vi "Nov_30.vi"() -> ()   [LabVIEW 2020]
uses:
  <vilib>/Analysis/3filter.llb/Filter Passband Type.ctl
  <vilib>/DAQmx/read.llb/DAQmx Read (Analog 1D DBL NChan 1Samp).vi
  <vilib>/DAQmx/create/channels.llb/DAQmx Create Channel (AI-Voltage-Basic).vi
  <vilib>/DAQmx/miscellaneous.llb/DAQmx Fill In Error Info.vi
  <vilib>/Analysis/3filter.llb/Butterworth Filter (DBL).vi
  <vilib>/Utility/file.llb/Write Delimited Spreadsheet (string).vi
  <vilib>/Utility/file.llb/Write Delimited Spreadsheet (DBL).vi
  <vilib>/Analysis/NI_AALBase.lvlib
panel:
  out "Force Plate":dynamicdata(graph)
  out "Swing":bool
  out "Accelerometers":dynamicdata(graph)
  out "Hit 1":bool
  out "Enlapsed Time (sec)":dbl
  in  "stop":bool
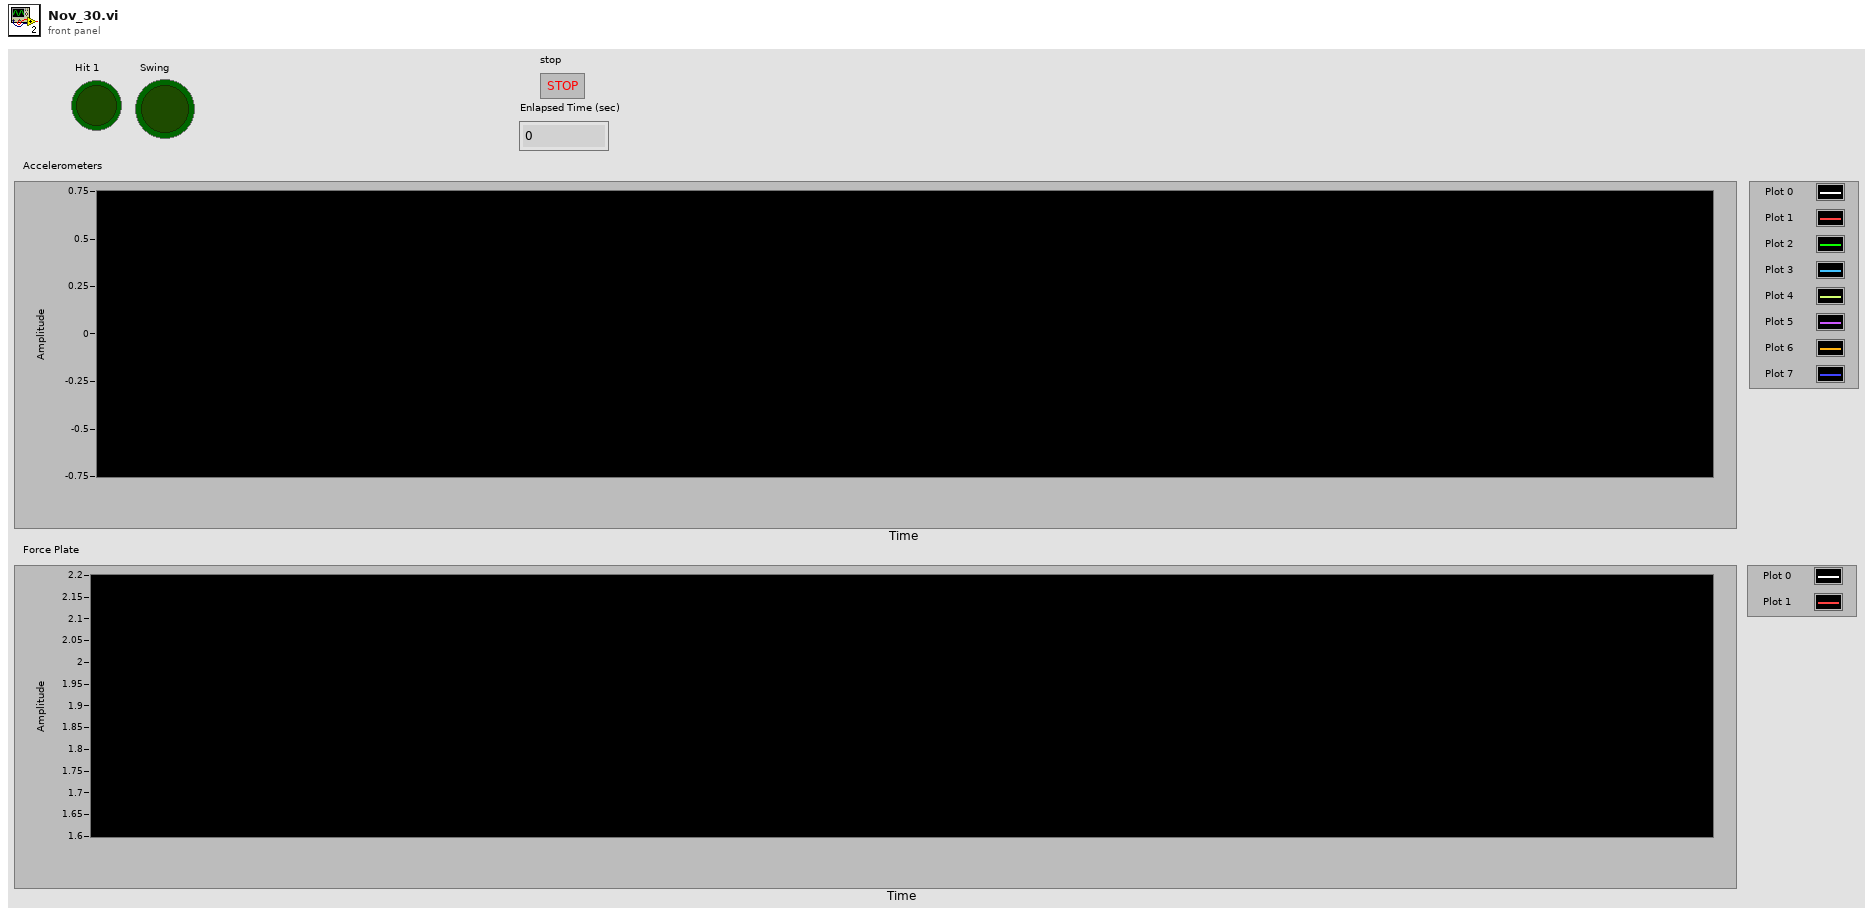
[diagram p1: front panel]
types:
  T1 = typedef "NI_AALBase.lvlib/Filter Passband Type.ctl" = enum32{"Lowpass", "Highpass", "Bandpass", "Bandstop"}
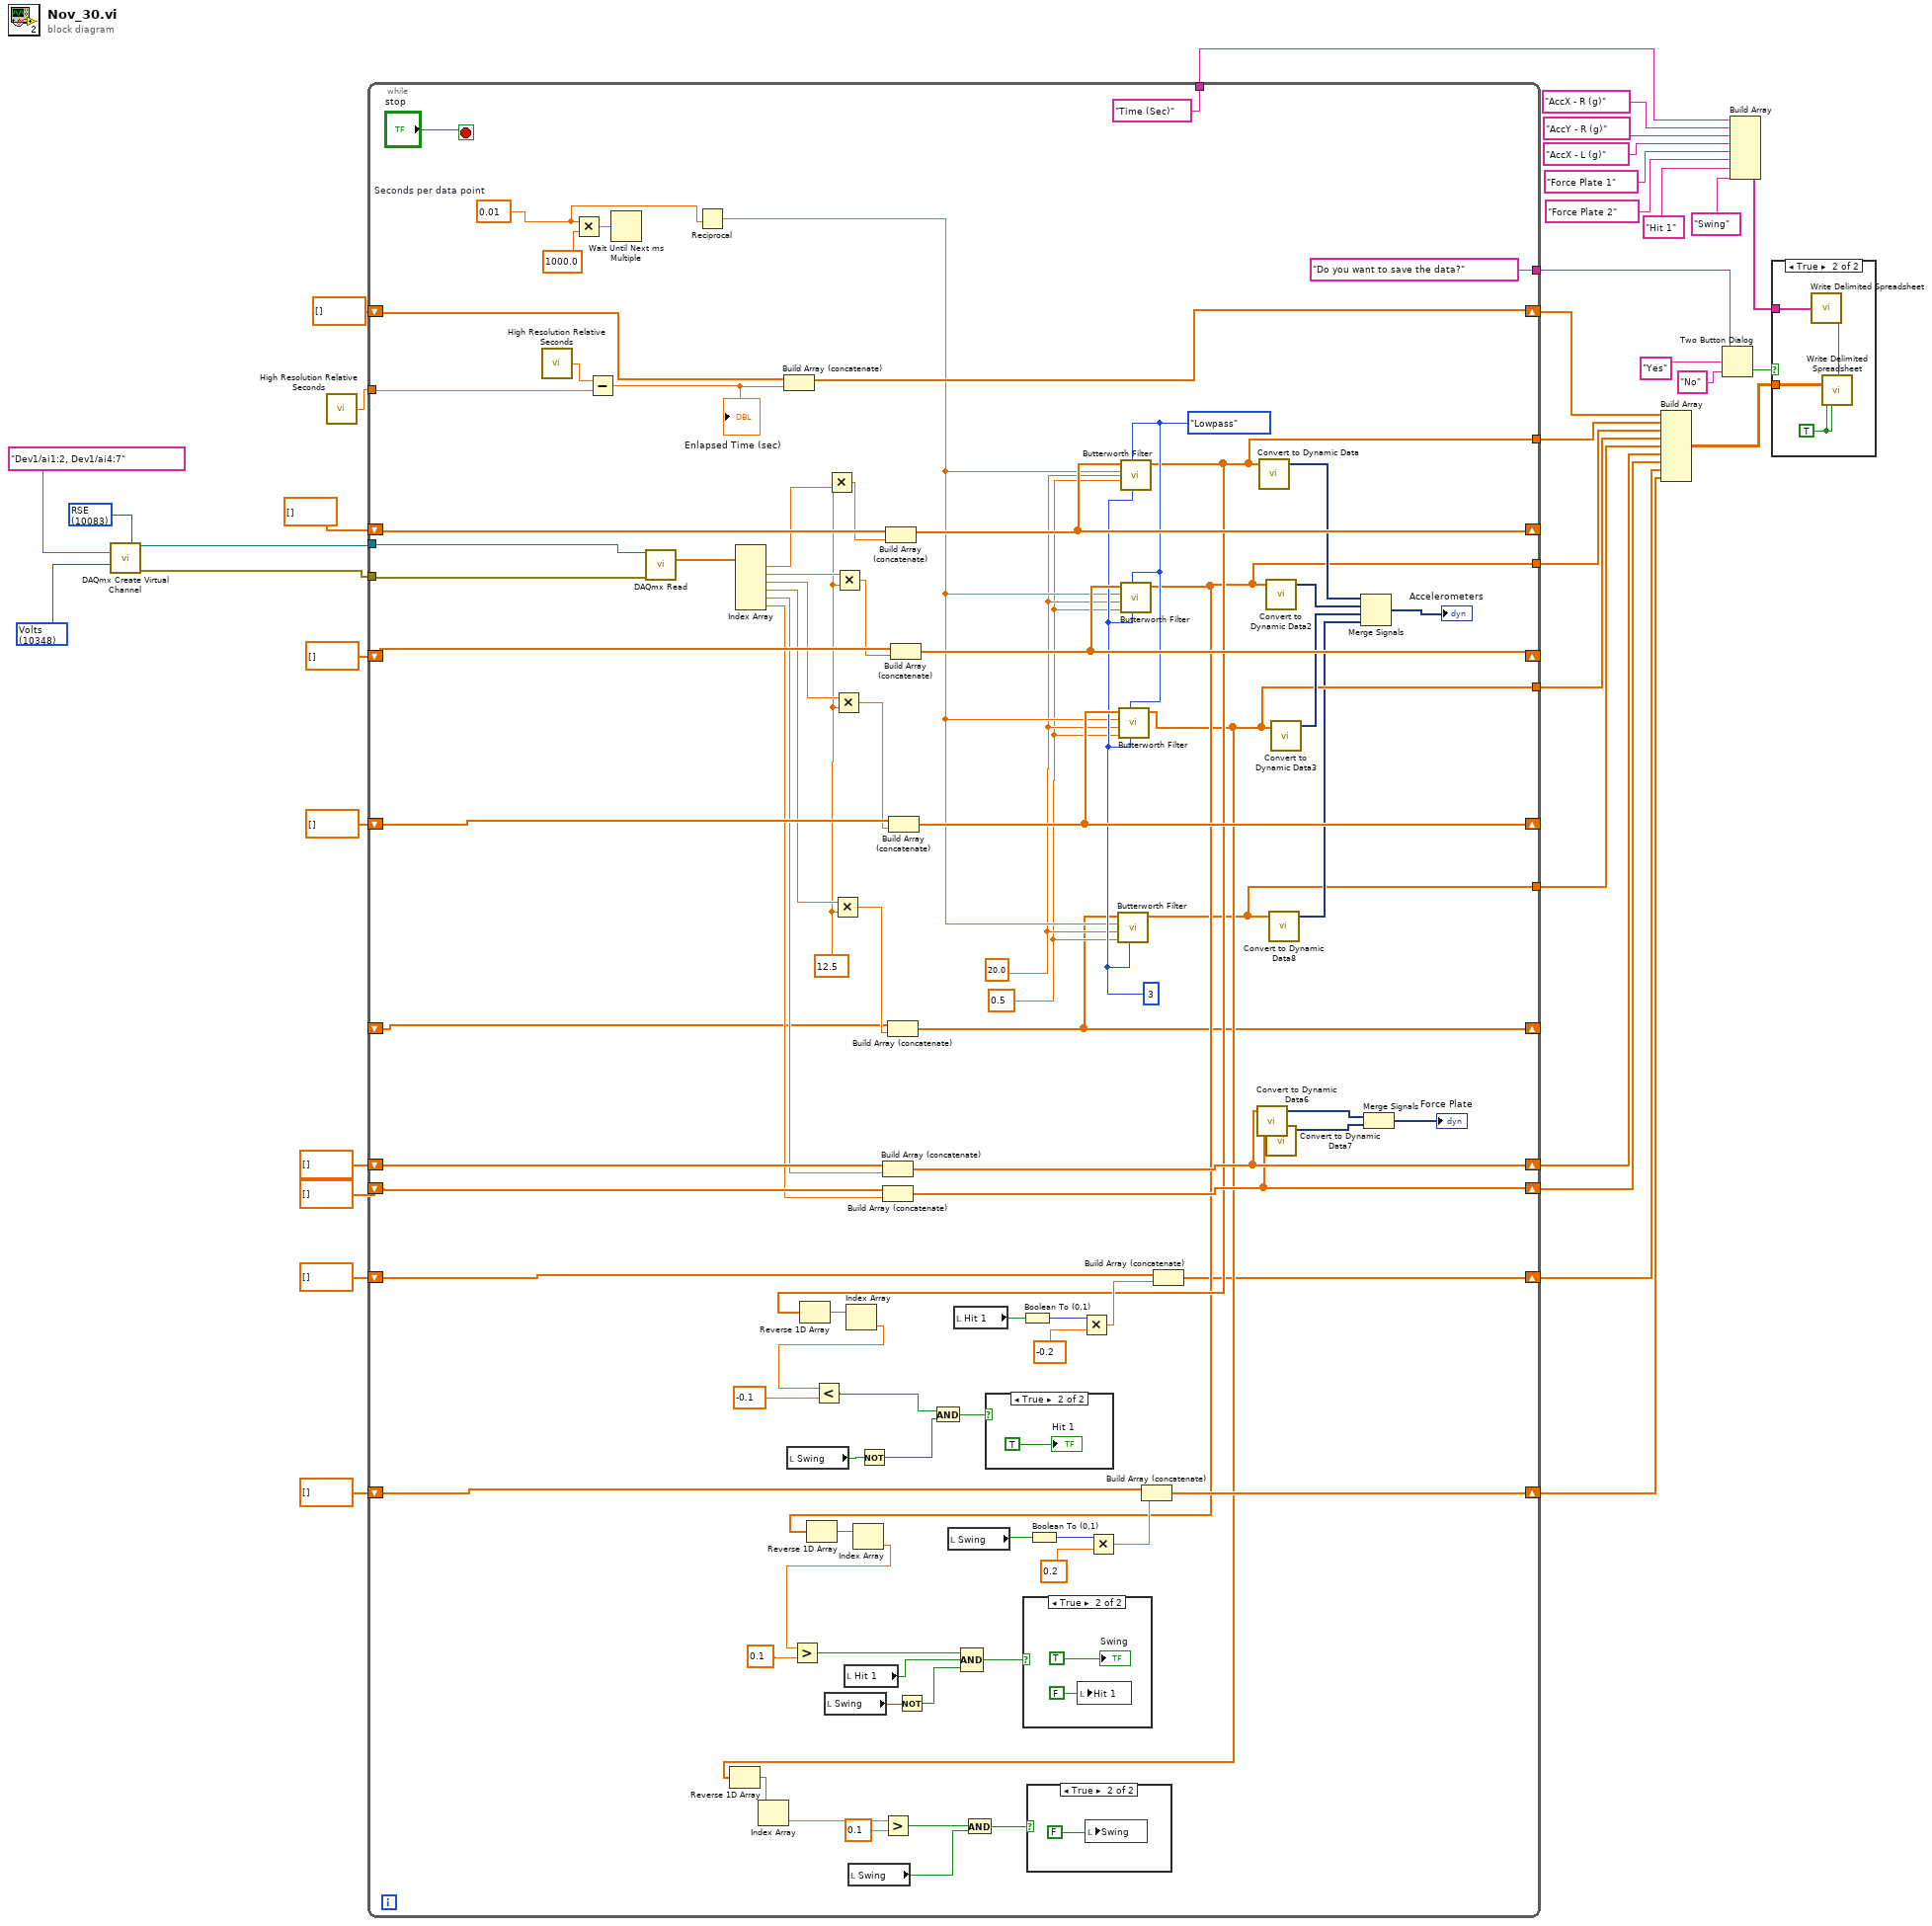
[diagram p0: block diagram]
diagram:
  w20 = 10348 items=["Volts"=10348, "From Custom Scale"=10065] ("units")
  w21 = 10083 items=["Default"=-1, "RSE"=10083, "NRSE"=10078, "Differential"=10106, "Pseudodifferential"=12529] ("input terminal configuration")
  n1 = call-poly <vilib>:"DAQmx Create Virtual Channel.vi"("input terminal configuration"=w21, "physical channels"=tag "Dev1/ai1:2, Dev1/ai4:7" ("Physical channels"), "units"=w20) -> ("task out"=w23:refnum<k21>, "error out"=w24:errorcluster)  [unwired: 11 in]
  n2 = call <vilib>:"High Resolution Relative Seconds.vi"() -> ("relative seconds"=w37:dbl)
  n3 = while {
    tunnel: w23 -> [w124]
    tunnel: w24 -> [w123]
    tunnel: w37 -> [w118]
    shift-right: [w83] -> w34
    shift-left: dbl[] [] -> [w116]
    shift-right: [w101] -> _
    shift-left: dbl[] [] -> [w114]
    shift-right: [w100] -> _
    shift-left: dbl[] [] -> [w113]
    tunnel: ["Time (Sec)"] -> w29
    tunnel: ["Do you want to save the data?" ("message")] -> w25
    shift-right: [w38] -> w4
    shift-left: dbl[] [] -> [w107]
    shift-right: [w79] -> w5
    shift-left: dbl[] [] -> [w90]
    shift-right: [w84] -> _
    shift-left: dbl[] [] -> [w87]
    shift-right: [w58] -> w2
    shift-left: dbl[] [] -> [w61]
    shift-right: [w56] -> w3
    shift-left: dbl[] [] -> [w60]
    tunnel: [w54] -> w8
    tunnel: [w53] -> w7
    tunnel: [w52] -> w6
    shift-right: [w41] -> _
    shift-left: _ -> [w40]
    tunnel: [w39] -> w1
    stop <- "stop" stop-if-true
    w48 = 3 ("order")
    w45 = 0.5 ("low cutoff freq: fl")
    w46 = 20.0 ("high cutoff freq: fh")
    w43 = 12.5 ("x")
    w62 = 0.01  # Seconds per data point
    w85 = Filter_Passband_Type."Lowpass" ("filter type")
    n4 = call <vilib>:"High Resolution Relative Seconds.vi"() -> ("relative seconds"=w119:dbl)
    n5 = Multiply(x=w62, y=1000.0) -> (x*y=w121:dbl)
    n6 = Subtract(x=w119, y=w118) -> (x-y=w117:dbl)
    "Enlapsed Time (sec)" <- w117
    n7 = Wait Until Next ms Multiple(millisecond multiple=w121) -> ()  [unwired: 1 out]
    n8 = call-poly <vilib>:"DAQmx Read.vi"("task/channels in"=w124, "error in"=w123) -> ("data"=w115:dbl[])  [unwired: 11 in, 2 out]
    n9 = Reciprocal(x=w62) -> (1/x=w47:dbl)
    n10 = Index Array(array=w115) -> (element #1=w110:dbl, element #2=w108:dbl, element #3=w88:dbl, element #4=w44:dbl, element #5=w50:dbl, element #6=w51:dbl)  [unwired: 6 in]
    n11 = Build Array (concatenate)(w116, w117) -> (w83:dbl[])
    n12 = local read "Swing"() -> (w73:bool)
    n13 = local read "Swing"() -> (w76:bool)
    n14 = Multiply(x=w43, y=w110) -> (x*y=w103:dbl)
    n15 = Multiply(x=w44, y=w43) -> (x*y=w49:dbl)
    n16 = Multiply(x=w88, y=w43) -> (x*y=w86:dbl)
    n17 = Multiply(x=w108, y=w43) -> (x*y=w109:dbl)
    n18 = local read "Hit 1"() -> (w77:bool)
    n19 = local read "Swing"() -> (w66:bool)
    n20 = Not(x=w73) -> (.not. x?=w72:bool)
    n21 = Build Array (concatenate)(w61, w50) -> (w58:dbl[])
    n22 = Build Array (concatenate)(w60, w51) -> (w56:dbl[])
    n23 = Build Array (concatenate)(w114, w103) -> (w101:dbl[])
    n24 = Build Array (concatenate)(w40, w49) -> (w41:dbl[])
    n25 = Build Array (concatenate)(w87, w86) -> (w84:dbl[])
    n26 = Build Array (concatenate)(w113, w109) -> (w100:dbl[])
    n27 = Not(x=w76) -> (.not. x?=w75:bool)
    n28 = local read "Swing"() -> (w89:bool)
    n29 = local read "Hit 1"() -> (w92:bool)
    n30 = Boolean To (0,1)(Boolean=w92) -> (0, 1=w105:i16)
    n31 = Boolean To (0,1)(Boolean=w89) -> (0, 1=w98:i16)
    n32 = Multiply(x=w105, y=-0.2) -> (x*y=w106:dbl)
    n33 = Multiply(x=w98, y=0.2) -> (x*y=w91:dbl)
    n34 = call-poly <vilib>:"Butterworth Filter.vi"("order"=w48, "low cutoff freq: fl"=w45, "high cutoff freq: fh"=w46, "sampling freq: fs"=w47, "X"=w41) -> ("Filtered X"=w39:dbl[])  [unwired: 3 in, 1 out]
    n35 = call-poly <vilib>:"Butterworth Filter.vi"("order"=w48, "filter type"=w85, "low cutoff freq: fl"=w45, "high cutoff freq: fh"=w46, "sampling freq: fs"=w47, "X"=w84) -> ("Filtered X"=w52:dbl[])  [unwired: 2 in, 1 out]
    n36 = Reverse 1D Array(array=w52) -> (reversed array=w64:dbl[])
    n37 = Index Array(array=w64) -> (element=w63:dbl)  [unwired: 1 in]
    n38 = Greater?(x=w63, y=0.1) -> (0:w65:bool)
    n39 = And(x=w65, y=w66) -> (x .and. y?=w67:bool)
    n40 = case shown="True" w67 {
      frame False {
      }
      frame True {
        n41 = local write "Swing"(FALSE) -> ()
      }
    }
    n42 = call-poly <vilib>:"Butterworth Filter.vi"("order"=w48, "filter type"=w85, "low cutoff freq: fl"=w45, "high cutoff freq: fh"=w46, "sampling freq: fs"=w47, "X"=w101) -> ("Filtered X"=w54:dbl[])  [unwired: 2 in, 1 out]
    n43 = Reverse 1D Array(array=w54) -> (reversed array=w102:dbl[])
    n44 = Index Array(array=w102) -> (element=w94:dbl)  [unwired: 1 in]
    n45 = Less?(x=w94, y=-0.1) -> (x < y?=w71:bool)
    n46 = And(x=w71, y=w72) -> (x .and. y?=w70:bool)
    n47 = case shown="True" w70 {
      frame False {
      }
      frame True {
        "Hit 1" <- TRUE
      }
    }
    n48 = call-poly <vilib>:"Butterworth Filter.vi"("order"=w48, "filter type"=w85, "low cutoff freq: fl"=w45, "high cutoff freq: fh"=w46, "sampling freq: fs"=w47, "X"=w100) -> ("Filtered X"=w53:dbl[])  [unwired: 2 in, 1 out]
    n49 = Reverse 1D Array(array=w53) -> (reversed array=w95:dbl[])
    n50 = Index Array(array=w95) -> (element=w96:dbl)  [unwired: 1 in]
    n51 = Greater?(x=w96, y=0.1) -> (0:w69:bool)
    n52 = Compound Arithmetic op=AND(w69, w77, w75) -> (w74:bool)
    n53 = case shown="True" w74 {
      frame False {
      }
      frame True {
        n54 = local write "Hit 1"(FALSE) -> ()
        "Swing" <- TRUE
      }
    }
    n55 = Build Array (concatenate)(w90, w91) -> (w79:dbl[])
    n56 = Build Array (concatenate)(w107, w106) -> (w38:dbl[])
    n57 = call "Convert to Dynamic Data6"("Array"=w58) -> ("Dynamic Data Type"=w57:dynamicdata)  [unwired: 3 in]
    n58 = call "Convert to Dynamic Data"("Array"=w54) -> ("Dynamic Data Type"=w82:dynamicdata)  [unwired: 3 in]
    n59 = call "Convert to Dynamic Data2"("Array"=w53) -> ("Dynamic Data Type"=w81:dynamicdata)  [unwired: 3 in]
    n60 = call "Convert to Dynamic Data7"("Array"=w56) -> ("Dynamic Data Type"=w55:dynamicdata)  [unwired: 3 in]
    n61 = call "Convert to Dynamic Data8"("Array"=w39) -> ("Dynamic Data Type"=w42:dynamicdata)  [unwired: 3 in]
    n62 = call "Convert to Dynamic Data3"("Array"=w52) -> ("Dynamic Data Type"=w80:dynamicdata)  [unwired: 3 in]
    n63 = Merge Signals(w82, w81, w80, w42) -> (→"Accelerometers":dynamicdata)
    n64 = Merge Signals(w57, w55) -> (→"Force Plate":dynamicdata)
  }
  n65 = Build Array(w34, w8, w7, w6, w1, w2, w3, w4, w5) -> (w33:dbl[][])
  n66 = Two Button Dialog(message=w25, 1:"No" ("F button name (\"Cancel\")"), 2:"Yes" ("T button name (\"OK\")")) -> (T button?=w28:bool)
  n67 = Build Array(w29, "AccX - R (g)", "AccY - R (g)", "AccX - L (g)", "Force Plate 1" ("element"), "Force Plate 2" ("element"), "Hit 1" ("element"), "Swing" ("element")) -> (w32:string[])
  n68 = case shown="True" w28 {
    tunnel: w33 -> [_ w132]
    tunnel: w32 -> [_ w131]
    frame False {
    }
    frame True {
      w130 = TRUE ("transpose? (no:F)")
      n69 = call-poly <vilib>:"Write Delimited Spreadsheet.vi"("1D data"=w131) -> ("new file path (Not A Path if cancelled)"=w129:path)  [unwired: 13 in, 1 out]
      n70 = call-poly <vilib>:"Write Delimited Spreadsheet.vi"("file path (dialog if empty)"=w129, "2D data"=w132, "append to file? (new file:F)"=w130, "transpose? (no:F)"=w130) -> ()  [unwired: 10 in, 2 out]
    }
  }
